vi "Timelapse viewer-Event handler-Load dataset.vi"(11 "queue":refnum<queue>) -> ()   [LabVIEW 2013]
uses:
  Typedefs/Speed Viewer States enum.ctl
  Globals/gl_Time series viewer globals.vi
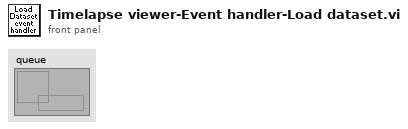
[diagram p1: front panel]
types:
  T1 = typedef "Speed Viewer States enum.ctl" = enum16{"Idle", "Initialise", "Playback", "Scroll bar event", "Speed cursor event", "Back to start", "Exit"}
  T2 = typedef "Timelapse viewer refs.ctl" = cluster{"This VI":refnum<vi>, "AVI Mode ind":refnum<vi>, "Play":refnum<vi>, "Stop":refnum<vi>, "Back":refnum<vi>, "Scrollbar":refnum<vi>, "Video length info":refnum<vi>, "Expected speed values":refnum<vi>, "Intensity":refnum<vi>, "Path":refnum<vi>, "Selection sliders":refnum<vi>, "Speed Graph ref":refnum<vi>, "Frame rate set (fps)":refnum<vi>}
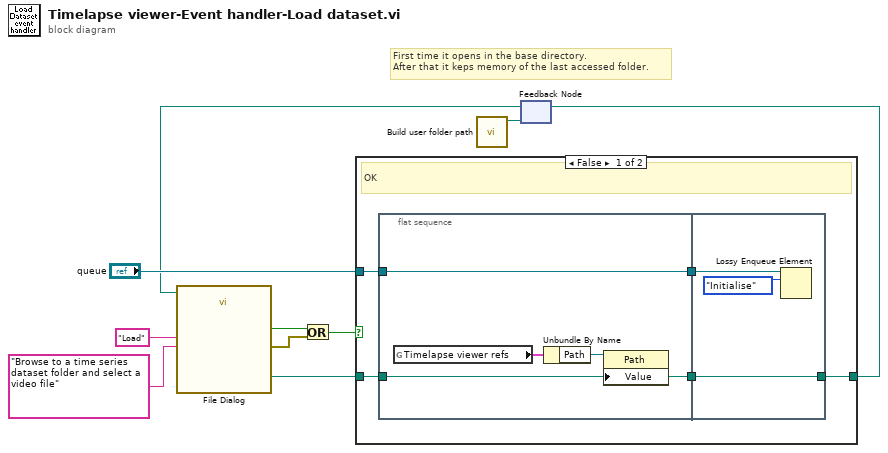
[diagram p0: block diagram]
diagram:
  # "First time it opens in the base directory.\nAfter that it keps memory of the last accessed folder."
  n1 = call "Build user folder path.vi"() -> ("Daily folder path with user folder appended?"=w1:path)  [unwired: 11 in]
  n2 = feedback #1(w1) -> (w5:path)
  n3 = call "File Dialog"("start path"=w5, "prompt"="Browse to a time series dataset folder and select a video file", "button label"="Load") -> ("selected path"=w10:path, "cancelled"=w7:bool, "error out"=w8:errorcluster)  [unwired: 9 in, 1 out]
  n4 = Or(x=w7, y=w8) -> (x .or. y?=w9:bool)
  n5 = case shown="False" w9 {
    tunnel: w10 -> [w15 w23]
    tunnel: "queue" -> [w13 _]
    tunnel: [w11 w23] -> w2
    frame False {
      # "OK"
      n6 = flat-sequence {
        tunnel: w15 -> [w16]
        tunnel: [w17] -> w14
        tunnel: w13 -> [w17]
        tunnel: [w16] -> w12
        tunnel: w14 -> [w21]
        tunnel: w12 -> [w20]
        tunnel: [w20] -> w11
        frame #0 {
          n7 = global read "gl_Time series viewer globals.vi" "Timelapse viewer refs"() -> (w19:T2)
          n8 = Unbundle By Name(w19) -> ("Path"=w18:refnum<vi>)
          n9 = property class="Path"(reference=w18, "Value"=w16) -> ()  [unwired: 1 in, 2 out]
        }
        frame #1 {
          n10 = Lossy Enqueue Element(queue=w21, element=Speed_Viewer_States_enum."Initialise" ("States")) -> ()  [unwired: 1 in, 4 out]
        }
      }
    }
    frame True {
      # "Error or cancelled"
    }
  }
  n11 = feedback-in #1(w2) -> ()
